vi "SaveOneImage (SubVI).vi"(7 "Save images path":path, 8 "error in (no error)":errorcluster, 9 "XYZ stage coordinates of image":dbl[](array[numeric]), 10 "Image Number":i32, 11 "Image":T1(plugin-control)) -> (0 "error out":errorcluster)   [LabVIEW 2016]
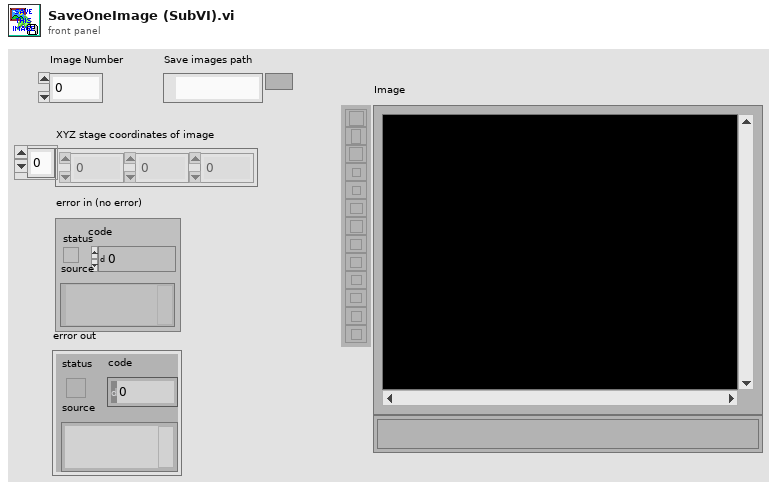
[diagram p1: front panel]
types:
  T1 = typedef "IMAQ Image.ctl" = refnum<image>
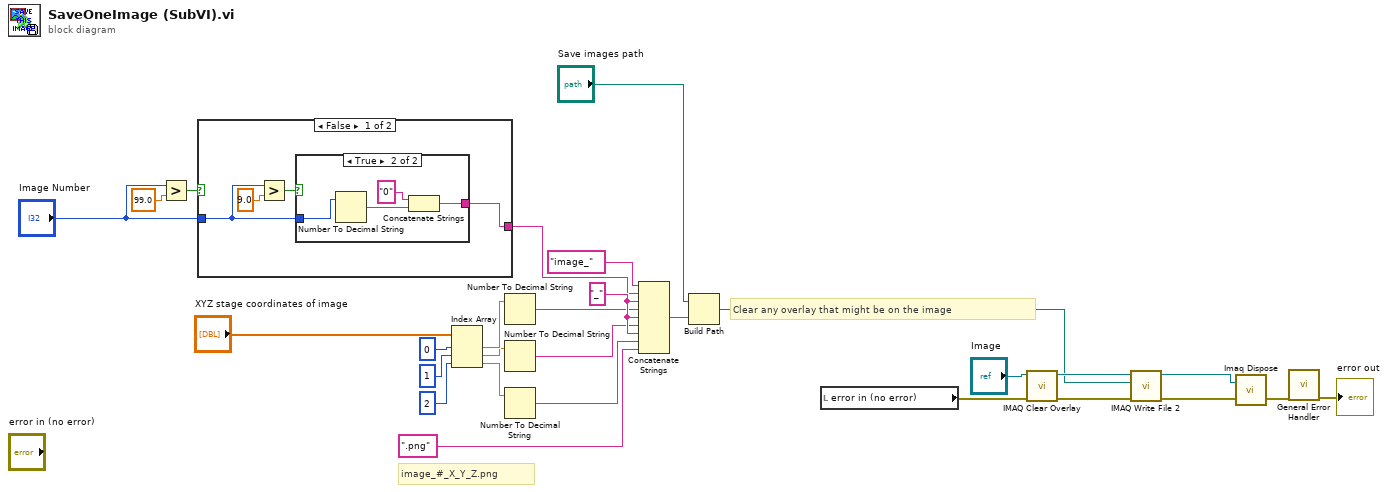
[diagram p0: block diagram]
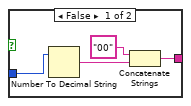
[diagram p2: hidden frame]
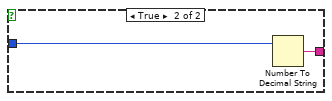
[diagram p3: hidden frame]
diagram:
  w19 = "_" ("string")
  # "image_#_X_Y_Z.png"
  # "Clear any overlay that might be on the image"
  n1 = Greater?(x="Image Number", y=99.0) -> (0:w14:bool)
  n2 = case shown="False" w14 {
    tunnel: "Image Number" -> [w29 w42]
    tunnel: [w31 w41] -> w18
    frame False {
      n3 = Greater?(x=w29, y=9.0) -> (0:w30:bool)
      n4 = case shown="True" w30 {
        tunnel: [w34 w37] -> w31
        tunnel: w29 -> [w33 w38]
        frame False {
          n5 = Number To Decimal String(number=w33) -> (decimal integer string=w36:string)  [unwired: 1 in]
          n6 = Concatenate Strings("00" ("string"), w36) -> (w34:string)
        }
        frame True {
          n7 = Number To Decimal String(number=w38) -> (decimal integer string=w40:string)  [unwired: 1 in]
          n8 = Concatenate Strings("0" ("string"), w40) -> (w37:string)
        }
      }
    }
    frame True {
      n9 = Number To Decimal String(number=w42) -> (decimal integer string=w41:string)  [unwired: 1 in]
    }
  }
  n10 = Index Array(array="XYZ stage coordinates of image", index #1=0 ("disabled index (col)"), index #2=1 ("disabled index (col)"), index #3=2 ("index (col)")) -> (element #1=w8:dbl, element #2=w4:dbl, element #3=w3:dbl)
  n11 = Number To Decimal String(number=w8) -> (decimal integer string=w17:string)  [unwired: 1 in]
  n12 = Number To Decimal String(number=w4) -> (decimal integer string=w16:string)  [unwired: 1 in]
  n13 = Number To Decimal String(number=w3) -> (decimal integer string=w15:string)  [unwired: 1 in]
  n14 = Concatenate Strings("image_" ("string"), w18, w19, w17, w19, w16, w19, w15, ".png" ("string")) -> (w28:string)
  n15 = Build Path(base path="Save images path", name or relative path=w28) -> (appended path=w21:path)
  n16 = local read "error in (no error)"() -> (w24:errorcluster)
  n17 = call "IMAQ Clear Overlay"("error in (no error)"=w24, "Image"="Image") -> ("error out"=w23:errorcluster, "Image Out"=w22:T1)  [unwired: 8 in]
  n18 = call-poly "IMAQ Write File 2"("error in (no error)"=w23, "File Path"=w21, "Image"=w22) -> ("error out"=w25:errorcluster, "Image Out (duplicate)"=w26:T1)  [unwired: 7 in]
  n19 = call "Imaq Dispose"("Image"=w26, "error in (no error)"=w25) -> ("error out"=w2:errorcluster)  [unwired: 4 in]
  n20 = call <vilib>:"General Error Handler.vi"("error in (no error)"=w2) -> ("error out"=→"error out":errorcluster)  [unwired: 10 in, 4 out]
